vi "Unflatten Packet.vi"(11 "Read Data":string) -> (0 "error out":errorcluster, 3 "Message Packet":variant)   [LabVIEW 2017, in "Network Logger Examples.lvlib" / "BasicNetworkProtocol.lvclass"]
uses:
  <vilib>/gpm_packages/@cs/event-logger/Examples/Examples/BasicNetworkProtocol/BasicNetworkProtocol.lvclass
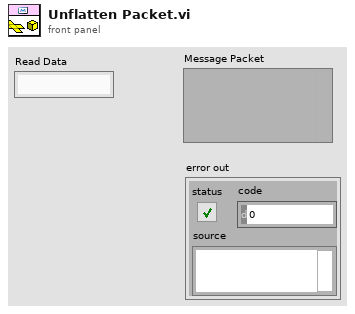
[diagram p1: front panel]
types:
  T1 = cluster{"type string":i16[], "data string":string}
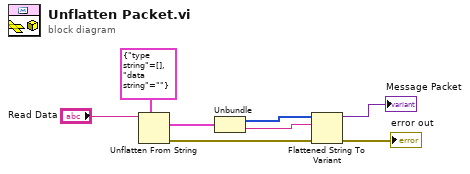
[diagram p0: block diagram]
diagram:
  n1 = Unflatten From String(type=T1 {"type string"=[], "data string"=""} ("output cluster"), binary string="Read Data") -> (value=w6:T1, error out=w5:errorcluster)  [unwired: 3 in, 1 out]
  n2 = Unbundle(w6) -> ("type string"=w3:i16[], "data string"=w2:string)
  n3 = Flattened String To Variant(4:w5, 6:w2, 7:w3) -> (0:→"error out":errorcluster, 3:→"Message Packet":variant)
